vi "Write Modulation queue.vi"(8 "error in (no error)":errorcluster, 10 "Modulation queue":refnum<queue>, 11 "Lock-in worker in":refnum<class "Lock-in worker.lvclass">) -> (0 "error out":errorcluster, 3 "Lock-in worker out":refnum<class "Lock-in worker.lvclass">)   [LabVIEW 2015, in "Lock-in worker.lvclass"]
uses:
  Lock-in worker.lvclass
  Lock-in modulation.ctl
  Lock-in worker.lvclass/Lock-in worker.ctl
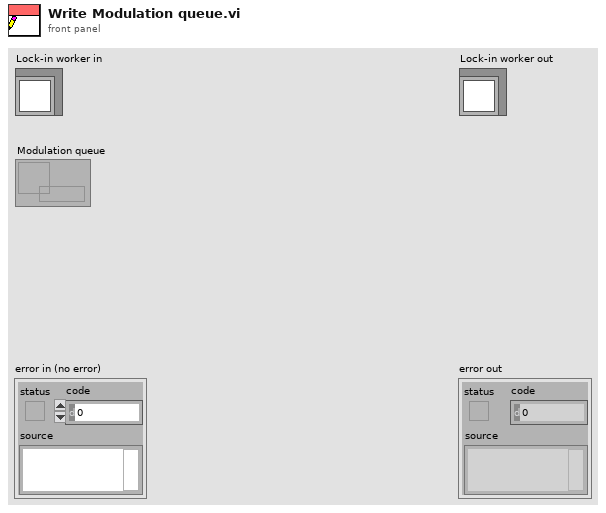
[diagram p1: front panel]
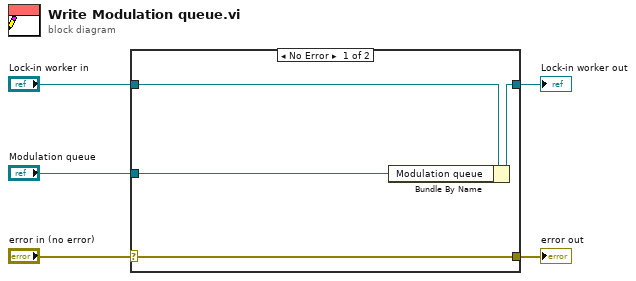
[diagram p0: block diagram]
diagram:
  n1 = case shown="No Error" "error in (no error)" {
    selector: "error in (no error)" -> [w9 w10]
    tunnel: [w9 w10] -> w4
    tunnel: [w7 w11] -> w2
    tunnel: "Lock-in worker in" -> [w8 w11]
    tunnel: "Modulation queue" -> [w6 _]
    frame No Error {
      n2 = Bundle By Name(cluster=w8, "Modulation queue"=w6) -> (w7:refnum<class "Lock-in worker.lvclass">)
    }
    frame Error {
    }
  }
  "error out" <- w4
  "Lock-in worker out" <- w2
